vi "Define PublicEvents Type.vi"(8 "error in (no error)":errorcluster, 11 "SMOFacade in":refnum<class "SMOFacade.lvclass">) -> (0 "error out":errorcluster, 2 "PublicEvents type":refnum<class "PublicEvents.lvclass">, 3 "SMOFacade out":refnum<class "SMOFacade.lvclass">)   [LabVIEW 2013, in "SMOFacade.lvclass"]
uses:
  SMOFacade.lvclass
  PublicEvents/PublicEvents.lvclass
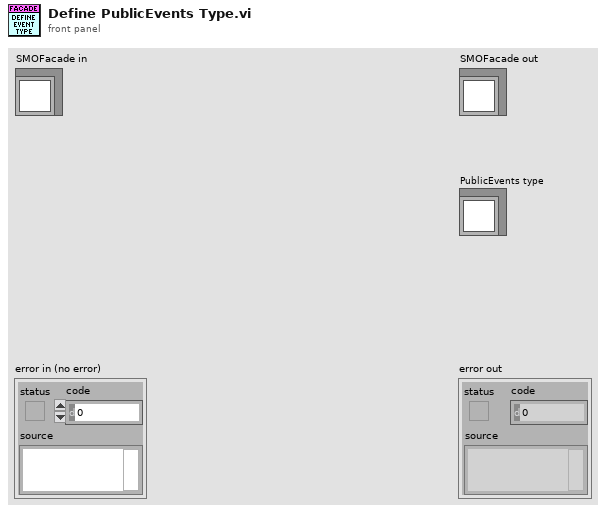
[diagram p1: front panel]
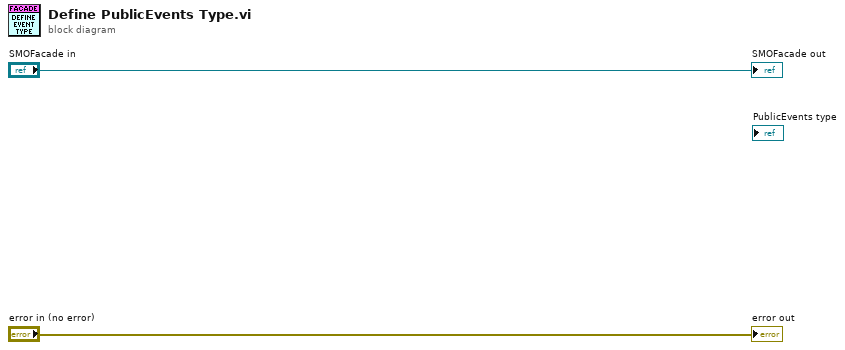
[diagram p0: block diagram]
diagram:
  "error out" <- "error in (no error)"
  "SMOFacade out" <- "SMOFacade in"
